vi "Index XYZ Trajectory v1.vi"(8 "Deform Array":dbl[](array[numeric])=[1.0, 1.0, 1.0, 0.0, 0.0, 0.0, 0.0, 0.0, 0.0], 9 "Pivot Pt":dbl[](array[numeric])=[0.0, 5.0, 0.0], 10 "Index":i32, 11 "Trajectory Cluster":T1) -> (1 "Indexed Cart Posit":dbl[](array[numeric]), 3 "Indexed XYZ Posit":dbl[](array[numeric]))   [LabVIEW 2016]
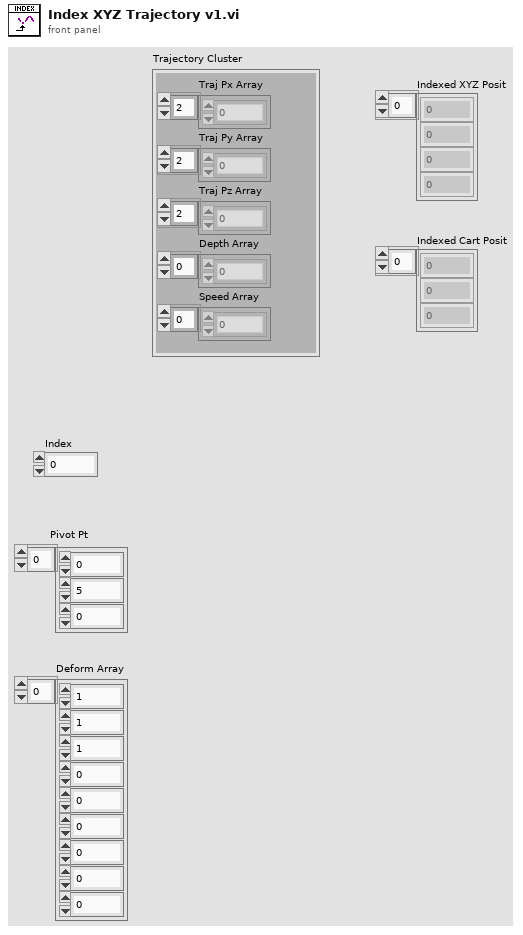
[diagram p1: front panel]
types:
  T1 = cluster{"Traj Px Array":dbl[], "Traj Py Array":dbl[], "Traj Pz Array":dbl[], "Speed Array":dbl[], "Depth Array":dbl[]}
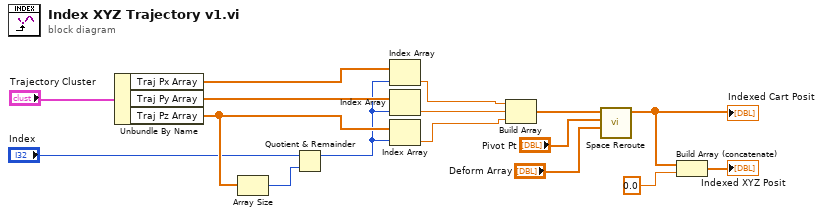
[diagram p0: block diagram]
diagram:
  n1 = Unbundle By Name("Trajectory Cluster") -> ("Traj Px Array"=w12:dbl[], "Traj Py Array"=w16:dbl[], "Traj Pz Array"=w10:dbl[])
  n2 = Array Size(array=w10) -> (size(s)=w9:i32)
  n3 = Quotient & Remainder(x="Index", y=w9) -> (x-y*floor(x/y)=w8:i32)  [unwired: 1 out]
  n4 = Index Array(array=w12, index=w8) -> (element=w15:dbl)
  n5 = Index Array(array=w16, index=w8) -> (element=w14:dbl)
  n6 = Index Array(array=w10, index=w8) -> (element=w13:dbl)
  n7 = Build Array(w15, w14, w13) -> (w6:dbl[])
  n8 = call "Space Reroute.vi"("Deform Array"="Deform Array", "Pivot Pt"="Pivot Pt", "Nominal Traj Pt"=w6) -> ("Reroute Traj Pt"=w1:dbl[])  [unwired: 8 in]
  "Indexed Cart Posit" <- w1
  n9 = Build Array (concatenate)(w1, 0.0 ("element")) -> (→"Indexed XYZ Posit":dbl[])
